vi "mcc_etc_open.vi"(8 "error in":errorcluster, 10 "units":i32(ring) items=["degC", "degF", "kelvin", "raw"], 11 "name":string="Dev1/Ti0:1") -> (0 "error out":errorcluster, 2 "status":bool=TRUE, 3 "task out":refnum<k24>)   [LabVIEW 2019]
uses:
  C:/Program Files (x86)/National Instruments/LabVIEW 2019/vi.lib/ULx/ULx_LV.dll
  Program Files (x86)/National Instruments/LabVIEW 2019/vi.lib/ULx/ULx_LV.dll
  <vilib>/ULx/Create Channel.llb/ULx Create Channel (AI-Temperature).vi
panel:
  in  "physical channels":refnum<k21>
  # "\"physical channels\" is used only to find available devices."
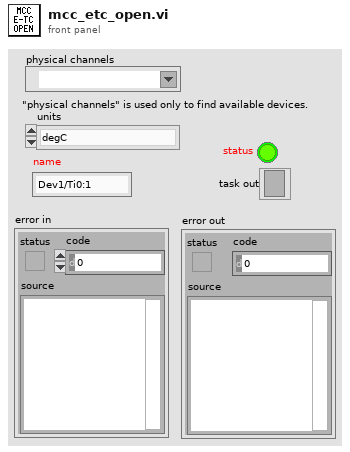
[diagram p1: front panel]
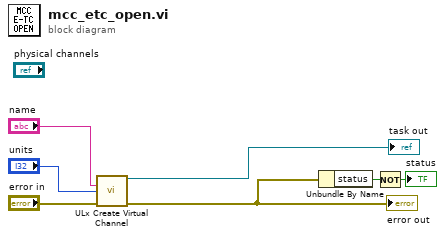
[diagram p0: block diagram]
diagram:
  n1 = call-poly <vilib>:"ULx Create Virtual Channel.vi"("physical channels"="name", "units"="units", "error in"="error in") -> ("task out"=→"task out":refnum<k24>, "error out"=w6:errorcluster)  [unwired: 11 in]
  "error out" <- w6
  n2 = Unbundle By Name(w6) -> ("status"=w2:bool)
  n3 = Not(x=w2) -> (.not. x?=→"status":bool)
